vi "Gobble.vi"(8 "error in (no error)":errorcluster, 11 "WildTurkey in":refnum<class "WildTurkey.lvclass">) -> (0 "error out":errorcluster, 2 "Gobble":string, 3 "WildTurkey out":refnum<class "WildTurkey.lvclass">)   [LabVIEW 2013, in "WildTurkey.lvclass"]
uses:
  WildTurkey.lvclass
  Turkey.lvclass/Turkey.lvclass
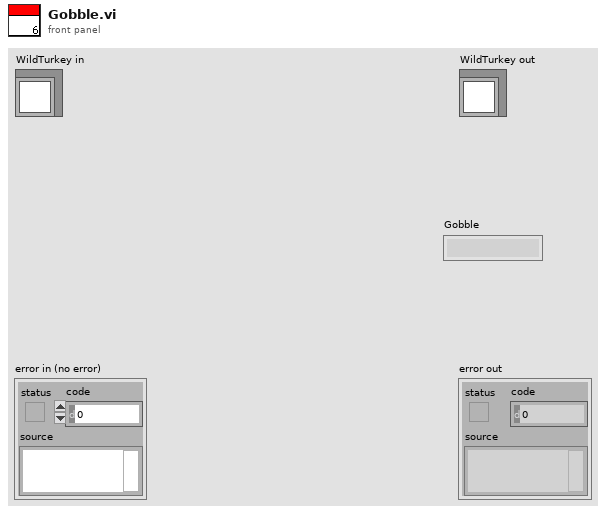
[diagram p1: front panel]
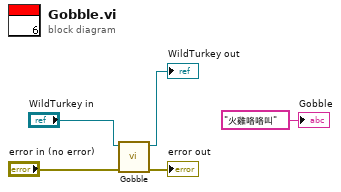
[diagram p0: block diagram]
diagram:
  n1 = call-parent "Gobble.vi"("error in (no error)"="error in (no error)", "Turkey in"="WildTurkey in") -> ("error out"=→"error out":errorcluster, "Turkey out"=→"WildTurkey out":refnum<class "WildTurkey.lvclass">)  [unwired: 7 in, 1 out]
  "Gobble" <- "火雞咯咯叫" ("Gobble")
